vi "stop or start VI by name.vi"(10 "stop (T) or start (F)":bool, 11 "VI name":string) -> (3 "VI is running":bool)   [LabVIEW 2012]
doc: "SciScan 1.2 160622"
panel:
  out "error out 4":errorcluster
  out "error out 3":errorcluster
  out "error out 2":errorcluster
  out "error out":errorcluster
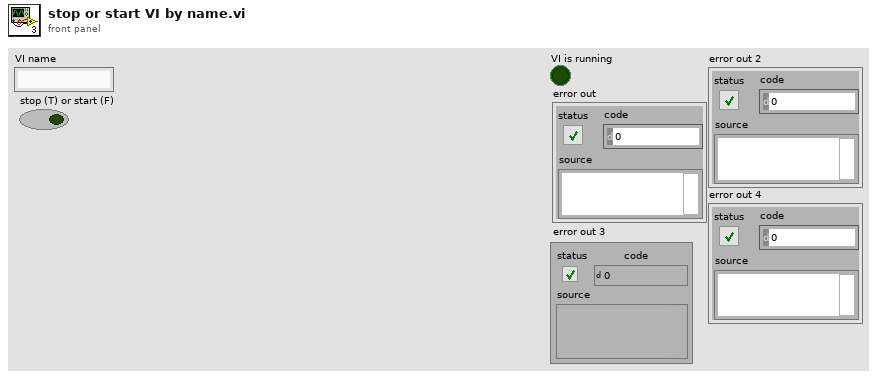
[diagram p1: front panel]
types:
  T1 = enum32{"Invalid", "Standard", "Closed", "Hidden", "Minimized", "Maximized"}
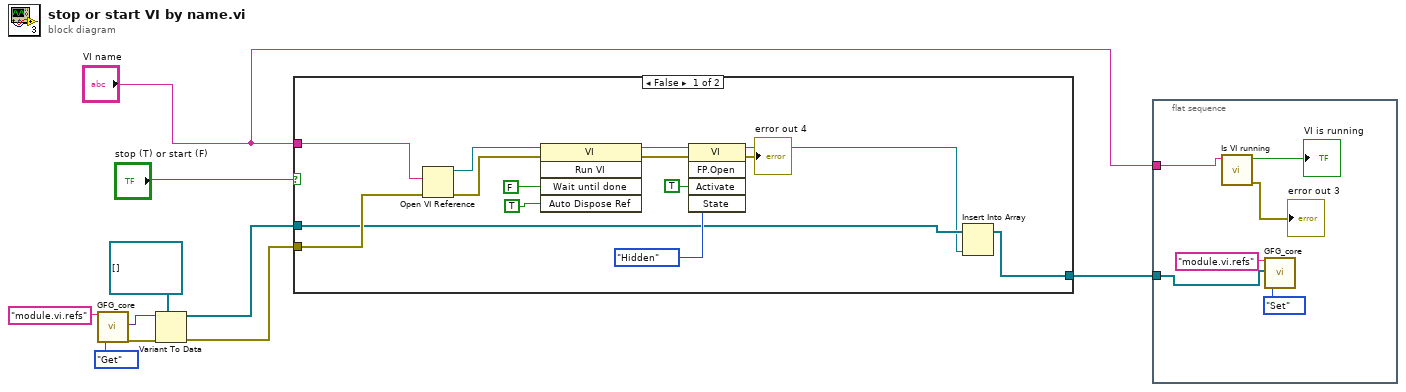
[diagram p0: block diagram]
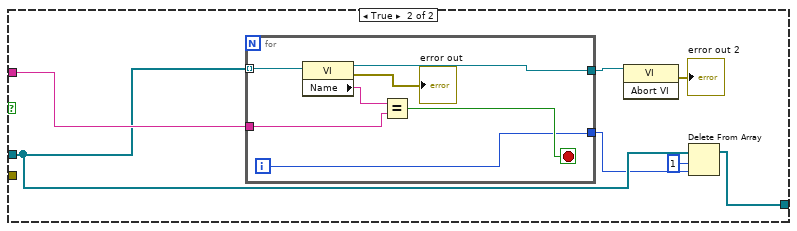
[diagram p2: hidden frame]
diagram:
  n1 = call "GFG_core.vi"("Variable Name in"="module.vi.refs", "Action"=enum16{"Init", "Set", "Get"}."Get") -> ("Variant Out"=w6:variant, "error out"=w8:errorcluster)  [unwired: 11 in, 5 out]
  n2 = Variant To Data(error in=w8, type=refnum<vi>[] [], Variant=w6) -> (data=w4:refnum<vi>[], error out=w5:errorcluster)
  n3 = case shown="False" "stop (T) or start (F)" {
    tunnel: "VI name" -> [w16 w31]
    tunnel: w5 -> [w15 _]
    tunnel: w4 -> [w14 w29]
    tunnel: [w13 w26] -> w3
    frame False {
      n4 = Open VI Reference(vi path=w16, error in (no error)=w15) -> (vi reference=w17:refnum<vi>, error out=w18:errorcluster)  [unwired: 4 in]
      n5 = invoke class="VI" method="Run VI"(reference=w17, error in=w18, "Wait until done"=FALSE, "Auto Dispose Ref"=TRUE ("Auto Dispose Reference")) -> (reference out=w23:refnum<vi>, error out=w19:errorcluster)  [unwired: 1 in, 3 out]
      n6 = invoke class="VI" method="FP.Open"(reference=w23, error in=w19, "Activate"=TRUE ("Activate?"), "State"=T1."Hidden") -> (reference out=w12:refnum<vi>, error out=→"error out 4":errorcluster)  [unwired: 1 in, 3 out]
      n7 = Insert Into Array(array=w14, new element=w12) -> (w13:refnum<vi>[])  [unwired: 1 in]
    }
    frame True {
      n8 = for {
        tunnel: w29 -> [w38] mode=indexing
        tunnel: w31 -> [w36]
        tunnel: [w34] -> w28
        tunnel: [w33] -> w30
        i -> [w34]
        stop <- w35 stop-if-true
        n9 = property class="VI"(reference=w38) -> (reference out=w33:refnum<vi>, error out=→"error out":errorcluster, "Name"=w37:string)  [unwired: 1 in]
        n10 = Equal?(x=w37, y=w36) -> (x = y?=w35:bool)
      }
      n11 = invoke class="VI" method="Abort VI"(reference=w30) -> (error out=→"error out 2":errorcluster)  [unwired: 2 in, 2 out]
      n12 = Delete From Array(array=w29, length=1, index=w28) -> (array with subset deleted=w26:refnum<vi>[])  [unwired: 1 out]
    }
  }
  n13 = flat-sequence {
    tunnel: w3 -> [w42]
    tunnel: "VI name" -> [w41]
    frame #0 {
      n14 = call "Is VI running.vi"("VI name"=w41) -> ("error out"=→"error out 3":errorcluster, "VI is running"=→"VI is running":bool)  [unwired: 9 in]
      n15 = call "GFG_core.vi"("Variable Name in"="module.vi.refs", "Variant in"=w42, "Action"=enum16{"Init", "Set", "Get"}."Set") -> ()  [unwired: 10 in, 7 out]
    }
  }
